vi "clone.vi"(0 "reference":refnum<class "CallEdge.lvclass">, 5 "error in (no error)":errorcluster) -> (14 "reference out":refnum<class "CallEdge.lvclass">, 15 "clonedEdge":refnum<class "AbstractEdge.lvclass">, 19 "error out":errorcluster)   [LabVIEW 2020, in "CallEdge.lvclass"]
doc: "Clone object"
uses:
  <resource>/Framework/Providers/Open_GDS/UML/CallEdge_class/CallEdge.lvclass
  C:/Program Files (x86)/National Instruments/LabVIEW 2020/resource/Framework/Providers/Open_GDS/UML/SegmentedLineEdge_class/SegmentedLineEdge.lvclass
  C:/Program Files (x86)/National Instruments/LabVIEW 2020/resource/Framework/Providers/Open_GDS/UML/GeneralPathEdge_class/GeneralPathEdge.lvclass
  C:/Program Files (x86)/National Instruments/LabVIEW 2020/resource/Framework/Providers/Open_GDS/UML/AbstractEdge_class/AbstractEdge.lvclass
  <resource>/Framework/Providers/Open_GDS/UML/AbstractEdge_class/AbstractEdge.lvclass
  <resource>/Framework/Providers/Open_GDS/UML/SegmentedLineEdge_class/SegmentedLineEdge.lvclass
  <resource>/Framework/Providers/Open_GDS/UML/GeneralPathEdge_class/GeneralPathEdge.lvclass
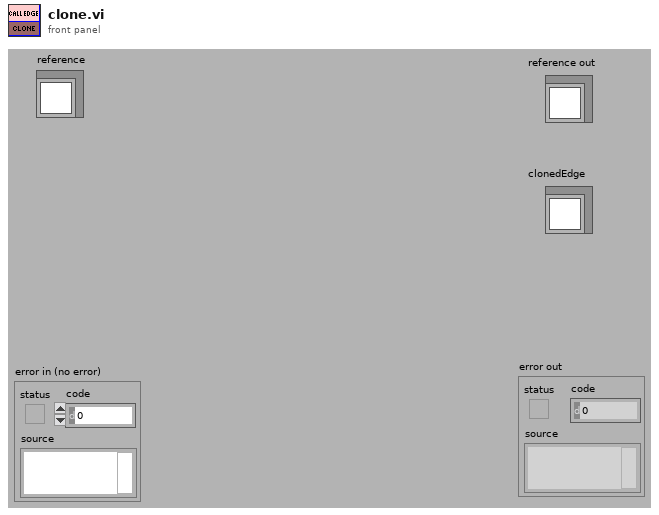
[diagram p1: front panel]
types:
  T1 = typedef "CallEdge.lvclass/ObjectAttributes.ctl" = cluster{"signal":bool}
  T2 = typedef "SegmentedLineEdge.lvclass/ObjectAttributes.ctl" = cluster{"lineStyle":refnum<class "LineStyle.lvclass">, "startArrowHead":refnum<class "ArrowHead.lvclass">, "endArrowHead":refnum<class "ArrowHead.lvclass">, "startLabel":string, "midLabel":string, "endLabel":string, "MidLabelOffset":T3, "SplitWire":bool}
  T3 = typedef "Point Point2D.ctl" = cluster{"x":dbl, "y":dbl}
  T4 = typedef "GeneralPathEdge.lvclass/ObjectAttributes.ctl" = cluster{"None":bool}
  T5 = typedef "AbstractEdge.lvclass/ObjectAttributes.ctl" = cluster{"start":refnum<class "AbstractNode.lvclass">, "end":refnum<class "AbstractNode.lvclass">}
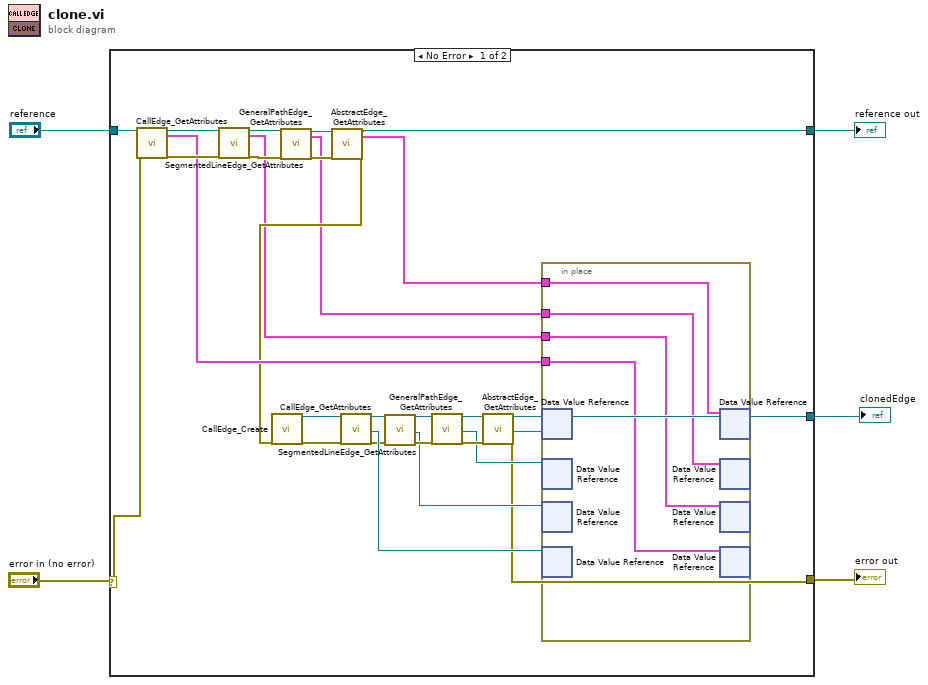
[diagram p0: block diagram]
diagram:
  n1 = case shown="No Error" "error in (no error)" {
    selector: "error in (no error)" -> [w32 w38]
    tunnel: "reference" -> [w33 w39]
    tunnel: [w7 w38] -> w4
    tunnel: [w12 w39] -> w1
    tunnel: [w8 _] -> w2
    frame No Error {
      n2 = call <resource>:"CallEdge_GetAttributes.vi"("reference in"=w33, "error in (no error)"=w32) -> ("reference out"=w29:refnum<class "CallEdge.lvclass">, "Data"=w17:T1, "error out"=w28:errorcluster)  [unwired: 1 in, 14 out]
      n3 = call <resource>:"SegmentedLineEdge_GetAttributes.vi"("reference in"=w29, "error in (no error)"=w28) -> ("reference out"=w6:refnum<class "CallEdge.lvclass">, "Data"=w11:T2, "error out"=w14:errorcluster)  [unwired: 14 in, 1 out]
      n4 = call <resource>:"GeneralPathEdge_GetAttributes.vi"("reference in"=w6, "error in (no error)"=w14) -> ("reference out"=w16:refnum<class "CallEdge.lvclass">, "Data"=w10:T4, "error out"=w15:errorcluster)  [unwired: 14 in, 1 out]
      n5 = call <resource>:"AbstractEdge_GetAttributes.vi"("reference in"=w16, "error in (no error)"=w15) -> ("reference out"=w12:refnum<class "CallEdge.lvclass">, "Data"=w9:T5, "error out"=w13:errorcluster)  [unwired: 14 in, 1 out]
      n6 = call <resource>:"CallEdge_Create.vi"("error in (no error)"=w13) -> ("reference out"=w30:refnum<class "CallEdge.lvclass">, "error out"=w31:errorcluster)  [unwired: 17 in]
      n7 = call <resource>:"CallEdge_GetAttributes.vi"("reference in"=w30, "error in (no error)"=w31) -> ("reference out"=w26:refnum<class "CallEdge.lvclass">, "DataRef"=w27:refnum<data-value>, "error out"=w21:errorcluster)  [unwired: 14 in, 1 out]
      n8 = call <resource>:"SegmentedLineEdge_GetAttributes.vi"("reference in"=w26, "error in (no error)"=w21) -> ("reference out"=w22:refnum<class "CallEdge.lvclass">, "DataRef"=w18:refnum<data-value>, "error out"=w25:errorcluster)  [unwired: 14 in, 1 out]
      n9 = call <resource>:"GeneralPathEdge_GetAttributes.vi"("reference in"=w22, "error in (no error)"=w25) -> ("reference out"=w23:refnum<class "CallEdge.lvclass">, "DataRef"=w19:refnum<data-value>, "error out"=w24:errorcluster)  [unwired: 14 in, 1 out]
      n10 = call <resource>:"AbstractEdge_GetAttributes.vi"("reference in"=w23, "error in (no error)"=w24) -> ("reference out"=w8:refnum<class "CallEdge.lvclass">, "DataRef"=w20:refnum<data-value>, "error out"=w7:errorcluster)  [unwired: 14 in, 1 out]
      n11 = in-place {
        in-place-border: w17 -> [w37]
        in-place-border: w11 -> [w36]
        in-place-border: w10 -> [w35]
        in-place-border: w9 -> [w34]
        n12 = in-place-dvr #1(w20) -> ()  [unwired: 2 out]
        n13 = in-place-dvr #2(w19) -> ()  [unwired: 2 out]
        n14 = in-place-dvr #3(w18) -> ()  [unwired: 2 out]
        n15 = in-place-dvr #4(w27) -> ()  [unwired: 2 out]
        n16 = in-place-dvr #1(w34) -> ()  [unwired: 2 out]
        n17 = in-place-dvr #2(w35) -> ()  [unwired: 2 out]
        n18 = in-place-dvr #3(w36) -> ()  [unwired: 2 out]
        n19 = in-place-dvr #4(w37) -> ()  [unwired: 2 out]
      }
    }
    frame Error {
    }
  }
  "reference out" <- w1
  "error out" <- w4
  "clonedEdge" <- w2
